vi "RSNRPZ Get Trigger Holdoff.vi"(8 "error in (no error)":errorcluster, 10 "Channel (1)":i32=1, 11 "VISA session":refnum<visa-resource-name> caption="VISA resource name") -> (0 "error out":errorcluster, 2 "Trigger Holdoff":dbl format="%.2p", 3 "dup VISA session":refnum<visa-resource-name> caption="VISA resource name")   [LabVIEW 2010]
doc: "This VI returns the value of a period after a trigger event within which all further trigger events are ignored.\n\nRemote-control command(s):\nTRIGger[1..4]:HOLDoff?"
uses:
  rsnrpz_32.dll
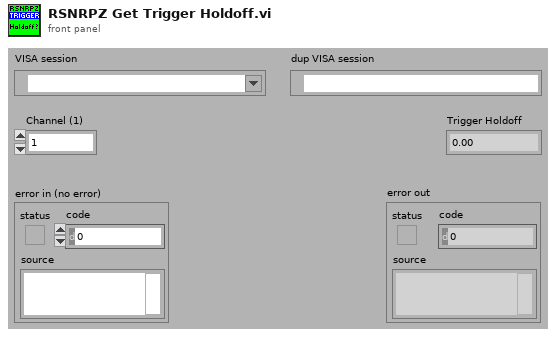
[diagram p1: front panel]
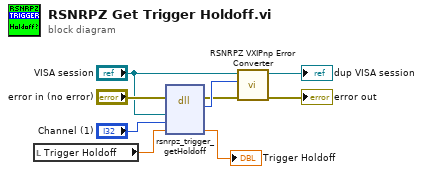
[diagram p0: block diagram]
diagram:
  n1 = local read "Trigger Holdoff"() -> (w7:dbl)
  n2 = dll-call lib="rsnrpz_32.dll" fn="rsnrpz_trigger_getHoldoff"(error in="error in (no error)", "VISA Session"="VISA session", "Channel"="Channel (1)", "Trigger Holdoff"=w7) -> (error out=w5:errorcluster, "Status"=w9:i32, "Trigger Holdoff"=→"Trigger Holdoff":dbl)  [unwired: 4 in, 1 out]
  n3 = call <instrlib>:"RSNRPZ VXIPnp Error Converter.vi"("error in"=w5, "VXIPnp error code"=w9, "VISA session"="VISA session") -> ("error out"=→"error out":errorcluster, "dup VISA session"=→"dup VISA session":refnum<visa-resource-name>)  [unwired: 7 in]
